vi "CaseStructure-Ver3-SlideControl.vi"() -> ()   [LabVIEW 2019]
panel:
  out "Less Than 7":bool
  out "Greater Than 7":bool
  out "Gauge":dbl(knob) scale=0.0..10.0
  in  "Slide":dbl(slide) scale=0.0..10.0
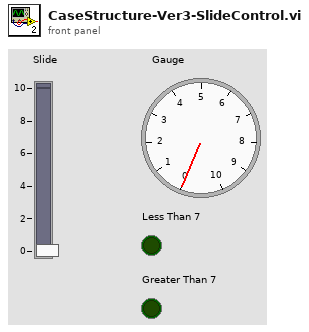
[diagram p1: front panel]
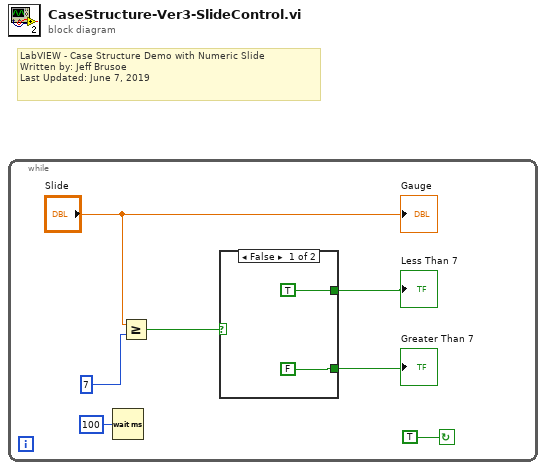
[diagram p0: block diagram]
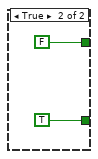
[diagram p2: hidden frame]
diagram:
  # "LabVIEW - Case Structure Demo with Numeric Slide\nWritten by: Jeff Brusoe\nLast Updated: June 7, 2019"
  n1 = while {
    stop <- TRUE continue-if-true
    n2 = Wait (ms)(milliseconds to wait=u32 100) -> ()  [unwired: 1 out]
    n3 = Greater Or Equal?(x="Slide", y=7) -> (x >= y?=w2:bool)
    n4 = case shown="False" w2 {
      tunnel: [TRUE FALSE] -> w4
      tunnel: [FALSE TRUE] -> w3
      frame False {
      }
      frame True {
      }
    }
    "Greater Than 7" <- w3
    "Less Than 7" <- w4
    "Gauge" <- "Slide"
  }
